vi "WILT Read From Spreadsheet File (string) with Prompt.vi"(4 "delimiter (\\t)":string="\t", 6 "transpose (no:F)":bool, 7 "format (%s)":string="%s", 8 "prompt":string="Choose file to read.", 9 "start of read offset (chars.:0)":i32, 10 "number of rows (all:-1)":i32=-1, 11 "file path (dialog if empty)":path) -> (0 "EOF?":bool, 1 "mark after read (chars.)":i32, 2 "first row":string[](array[string]), 3 "all rows":string[][](array[string]), 5 "new file path (Not A Path if cancelled)":path)   [LabVIEW 2016]
doc: "Reads a specified number of lines or rows from a numeric text file beginning at a specified character offset and converts the data to a 2D, double-precision array of numbers, strings, or integers. You must manually select the polymorphic instance you want to use."
panel:
  in  "type (empty)":string[][](array[string])
  in  "max characters/row  (no limit:0)":i32
  # "row\ncolumn"
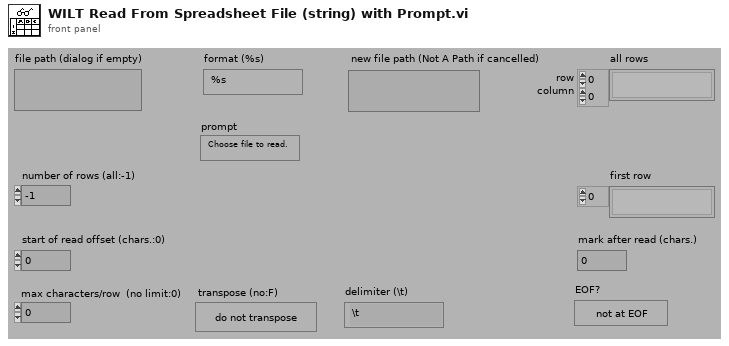
[diagram p1: front panel]
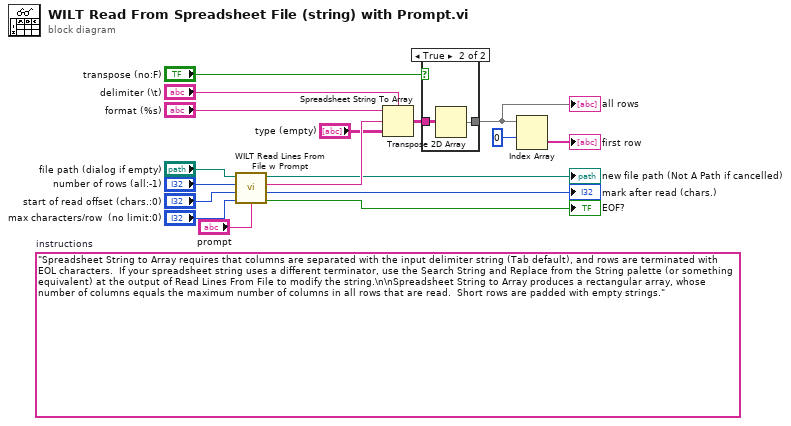
[diagram p0: block diagram]
diagram:
  (unwired) "Spreadsheet String to Array requires that columns are separated with the input delimiter string (Tab default), and rows are terminated with EOL characters.  If your spreadsheet string uses a different terminator, use the Search String and Replace from the String palette (or something equivalent) at the output of Read Lines From File to modify the string.\n\nSpreadsheet String to Array produces a rectangular array, whose number of columns equals the maximum number of columns in all rows that are read.  Short rows are padded with empty strings."  # instructions
  n1 = call "WILT Read Lines From File w Prompt.vi"("file path (dialog if empty)"="file path (dialog if empty)", "number of lines (all:-1)"="number of rows (all:-1)", "prompt"="prompt", "start of read offset (chars.:0)"="start of read offset (chars.:0)", "[max characters per line]  (no limit:0)"="max characters/row  (no limit:0)") -> ("new file path (Not A Path if cancelled)"=→"new file path (Not A Path if cancelled)":path, "line string"=w13:string, "mark after read (chars.)"=→"mark after read (chars.)":i32, "EOF?"=→"EOF?":bool)  [unwired: 1 in]
  n2 = Spreadsheet String To Array(delimiter (Tab)="delimiter (\\t)", format string="format (%s)", spreadsheet string=w13, array type (2D Dbl)="type (empty)") -> (array=w4:string[][])
  n3 = case shown="True" "transpose (no:F)" {
    tunnel: w4 -> [w18 w20]
    tunnel: [w18 w19] -> w2
    frame False {
    }
    frame True {
      n4 = Transpose 2D Array(2D array=w20) -> (transposed array=w19:string[][])
    }
  }
  "all rows" <- w2
  n5 = Index Array(array=w2, index (row)=0) -> (element=→"first row":string[])  [unwired: 1 in]
